vi "파일전송클라이언트.vi"() -> ()   [LabVIEW 2018]
panel:
  out "Sever Connected":bool
  in  "Folder Path":path=path "E:/images" caption="다운로드  경로"
  in  "다운로드":bool
  out "선택한 파일":string
  in  "파일 리스트":i32(listbox)=-1
  in  "업데이트":bool
  out "Echo":string
  in  "정지":bool
  in  "데이터 입력":string
  in  "전송":bool
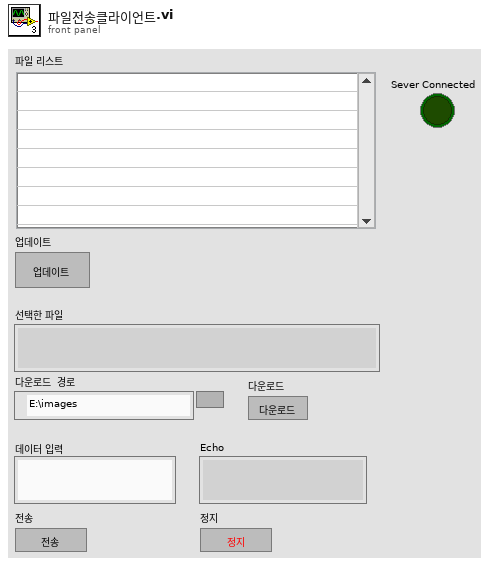
[diagram p1: front panel]
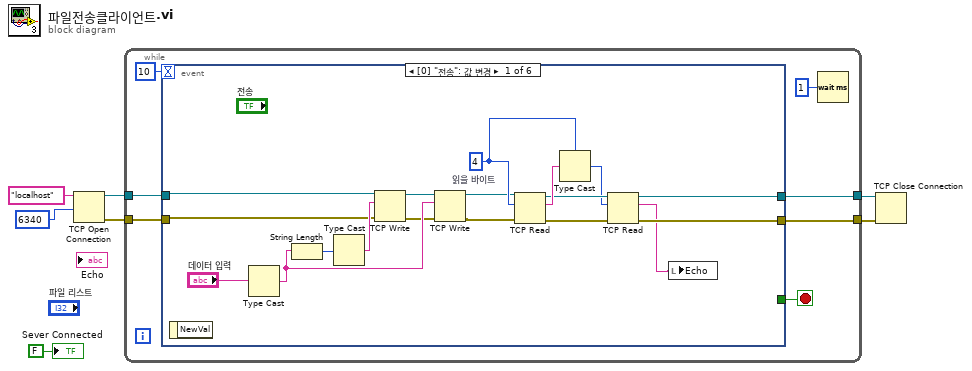
[diagram p0: block diagram]
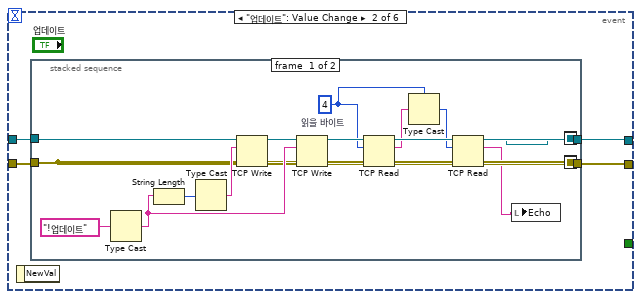
[diagram p2: hidden frame]
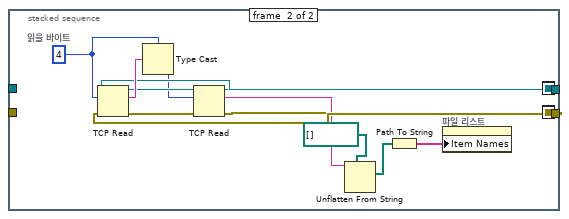
[diagram p3: hidden frame]
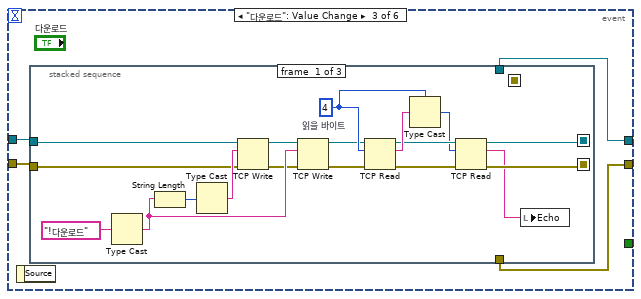
[diagram p4: hidden frame]
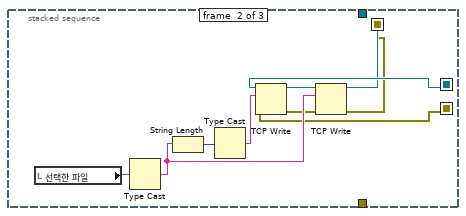
[diagram p5: hidden frame]
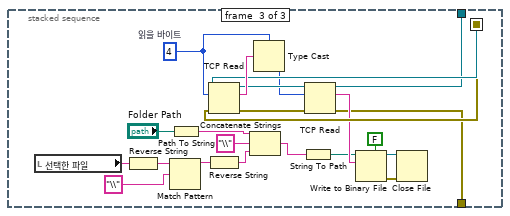
[diagram p6: hidden frame]
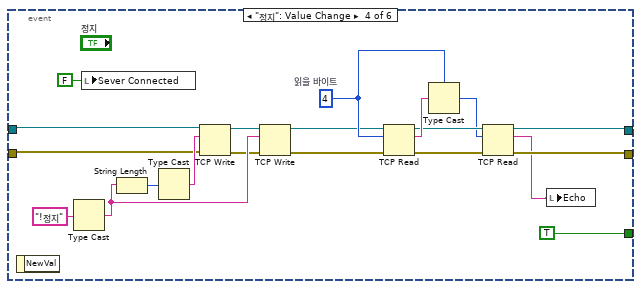
[diagram p7: hidden frame]
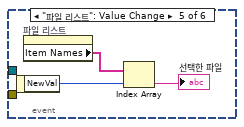
[diagram p8: hidden frame]
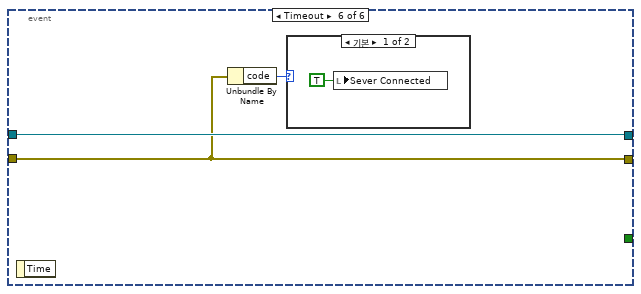
[diagram p9: hidden frame]
diagram:
  n1 = TCP Open Connection(address="localhost" ("주소"), remote port or service name=u16 6340 ("포트")) -> (connection ID=w5:refnum<k5>, error out=w3:errorcluster)  [unwired: 3 in]
  n2 = while {
    tunnel: w5 -> [w14]
    tunnel: [w12] -> w4
    tunnel: w3 -> [w13]
    tunnel: [w11] -> w2
    stop <- w10 stop-if-true
    n3 = event shown="[0] \"전송\": 값 변경" {
      selector: _ -> [_ _ _ _ _ _]
      dyn-events: _ -> [_ _ _ _ _ _]
      timeout: 10 -> [_ _ _ _ _ _]
      tunnel: w14 -> [w26 w36 w71 w137 _ w148]
      tunnel: w13 -> [w25 w35 w70 w136 _ w147]
      tunnel: [w17 w34 w69 w128 _ w148] -> w12
      tunnel: [w16 w33 w68 w127 _ w147] -> w11
      tunnel: [_ _ _ TRUE _ _] -> w10
      event "전송": Value Change {
        w23 = 4  # 읽을 바이트
        n4 = event-data() -> ()  [unwired: 1 in, 1 out]
        n5 = Type Cast(x="데이터 입력") -> (*(type *) &x=w30:string)  [unwired: 1 in]
        n6 = String Length(string=w30) -> (length=w31:i32)
        n7 = Type Cast(x=w31) -> (*(type *) &x=w32:string)  [unwired: 1 in]
        n8 = TCP Write(connection ID=w26, data in=w32, error in (no error)=w25) -> (connection ID out=w29:refnum<k5>, error out=w27:errorcluster)  [unwired: 1 in, 1 out]
        n9 = TCP Write(connection ID=w29, data in=w30, error in (no error)=w27) -> (connection ID out=w22:refnum<k5>, error out=w21:errorcluster)  [unwired: 1 in, 1 out]
        n10 = TCP Read(connection ID=w22, bytes to read=w23, error in (no error)=w21) -> (connection ID out=w19:refnum<k5>, data out=w24:string, error out=w20:errorcluster)  [unwired: 2 in]
        n11 = Type Cast(type=w23, x=w24) -> (*(type *) &x=w18:i32)
        n12 = TCP Read(connection ID=w19, bytes to read=w18, error in (no error)=w20) -> (connection ID out=w17:refnum<k5>, data out=w15:string, error out=w16:errorcluster)  [unwired: 2 in]
        n13 = local write "Echo"(w15) -> ()
      }
      event "업데이트": Value Change {
        n14 = event-data() -> ()  [unwired: 1 in, 1 out]
        n15 = stacked-sequence {
          seq-local: [w49 _] -> [_ w65]
          seq-local: [w48 _] -> [_ w64]
          seq-local: [w40 _] -> [_ _]
          seq-local: [w39 _] -> [_ _]
          tunnel: w36 -> [w49 _]
          tunnel: w35 -> [w48 _]
          tunnel: [_ w58] -> w34
          tunnel: [_ w57] -> w33
          frame #0 {
            w46 = 4  # 읽을 바이트
            n16 = Type Cast(x="!업데이트") -> (*(type *) &x=w52:string)  [unwired: 1 in]
            n17 = String Length(string=w52) -> (length=w53:i32)
            n18 = Type Cast(x=w53) -> (*(type *) &x=w54:string)  [unwired: 1 in]
            n19 = TCP Write(connection ID=w49, data in=w54, error in (no error)=w48) -> (connection ID out=w51:refnum<k5>, error out=w50:errorcluster)  [unwired: 1 in, 1 out]
            n20 = TCP Write(connection ID=w51, data in=w52, error in (no error)=w50) -> (connection ID out=w45:refnum<k5>, error out=w44:errorcluster)  [unwired: 1 in, 1 out]
            n21 = TCP Read(connection ID=w45, bytes to read=w46, error in (no error)=w44) -> (connection ID out=w42:refnum<k5>, data out=w47:string, error out=w43:errorcluster)  [unwired: 2 in]
            n22 = Type Cast(type=w46, x=w47) -> (*(type *) &x=w41:i32)
            n23 = TCP Read(connection ID=w42, bytes to read=w41, error in (no error)=w43) -> (connection ID out=w40:refnum<k5>, data out=w38:string, error out=w39:errorcluster)  [unwired: 2 in]
            n24 = local write "Echo"(w38) -> ()
          }
          frame #1 {
            w66 = 4  # 읽을 바이트
            n25 = TCP Read(connection ID=w65, bytes to read=w66, error in (no error)=w64) -> (connection ID out=w60:refnum<k5>, data out=w67:string, error out=w59:errorcluster)  [unwired: 2 in]
            n26 = Type Cast(type=w66, x=w67) -> (*(type *) &x=w55:i32)
            n27 = TCP Read(connection ID=w60, bytes to read=w55, error in (no error)=w59) -> (connection ID out=w58:refnum<k5>, data out=w62:string, error out=w57:errorcluster)  [unwired: 2 in]
            n28 = Unflatten From String(type=path[] [], binary string=w62) -> (value=w63:path[])  [unwired: 3 in, 2 out]
            n29 = Path To String(path=w63) -> (string=w56:string[])
            n30 = property on="파일 리스트" class="LstBox (엄격한)"("Item Names"=w56) -> ()  [unwired: 2 in, 2 out]
          }
        }
      }
      event "다운로드": Value Change {
        n31 = event-data() -> ()  [unwired: 1 in, 1 out]
        n32 = stacked-sequence {
          seq-local: [w77 _ _] -> [_ w93 _]
          seq-local: [w76 _ _] -> [_ w92 _]
          seq-local: [_ w91 _] -> [_ _ w120]
          seq-local: [_ w90 _] -> [_ _ w119]
          tunnel: w71 -> [w73 _ _]
          tunnel: w70 -> [w72 _ _]
          tunnel: [_ _ w111] -> w69
          tunnel: [_ _ w110] -> w68
          frame #0 {
            w83 = 4  # 읽을 바이트
            n33 = Type Cast(x="!다운로드") -> (*(type *) &x=w87:string)  [unwired: 1 in]
            n34 = String Length(string=w87) -> (length=w88:i32)
            n35 = Type Cast(x=w88) -> (*(type *) &x=w89:string)  [unwired: 1 in]
            n36 = TCP Write(connection ID=w73, data in=w89, error in (no error)=w72) -> (connection ID out=w86:refnum<k5>, error out=w85:errorcluster)  [unwired: 1 in, 1 out]
            n37 = TCP Write(connection ID=w86, data in=w87, error in (no error)=w85) -> (connection ID out=w82:refnum<k5>, error out=w81:errorcluster)  [unwired: 1 in, 1 out]
            n38 = TCP Read(connection ID=w82, bytes to read=w83, error in (no error)=w81) -> (connection ID out=w79:refnum<k5>, data out=w84:string, error out=w80:errorcluster)  [unwired: 2 in]
            n39 = Type Cast(type=w83, x=w84) -> (*(type *) &x=w78:i32)
            n40 = TCP Read(connection ID=w79, bytes to read=w78, error in (no error)=w80) -> (connection ID out=w77:refnum<k5>, data out=w74:string, error out=w76:errorcluster)  [unwired: 2 in]
            n41 = local write "Echo"(w74) -> ()
          }
          frame #1 {
            n42 = local read "선택한 파일"() -> (w94:string)
            n43 = Type Cast(x=w94) -> (*(type *) &x=w97:string)  [unwired: 1 in]
            n44 = String Length(string=w97) -> (length=w98:i32)
            n45 = Type Cast(x=w98) -> (*(type *) &x=w99:string)  [unwired: 1 in]
            n46 = TCP Write(connection ID=w93, data in=w99, error in (no error)=w92) -> (connection ID out=w96:refnum<k5>, error out=w95:errorcluster)  [unwired: 1 in, 1 out]
            n47 = TCP Write(connection ID=w96, data in=w97, error in (no error)=w95) -> (connection ID out=w91:refnum<k5>, error out=w90:errorcluster)  [unwired: 1 in, 1 out]
          }
          frame #2 {
            w121 = 4  # 읽을 바이트
            n48 = local read "선택한 파일"() -> (w107:string)
            n49 = Reverse String(1:w107) -> (0:w106:string)
            n50 = Match Pattern(string=w106, regular expression="\\" ("정규식")) -> (before substring=w108:string)  [unwired: 1 in, 3 out]
            n51 = Path To String(path="Folder Path") -> (string=w100:string)
            n52 = TCP Read(connection ID=w120, bytes to read=w121, error in (no error)=w119) -> (connection ID out=w118:refnum<k5>, data out=w122:string, error out=w117:errorcluster)  [unwired: 2 in]
            n53 = Reverse String(1:w108) -> (0:w104:string)
            n54 = Concatenate Strings(w100, "\\" ("문자열"), w104) -> (w101:string)
            n55 = Type Cast(type=w121, x=w122) -> (*(type *) &x=w116:i32)
            n56 = String To Path(string=w101) -> (path=w102:path)
            n57 = TCP Read(connection ID=w118, bytes to read=w116, error in (no error)=w117) -> (connection ID out=w111:refnum<k5>, data out=w112:string, error out=w110:errorcluster)  [unwired: 2 in]
            n58 = Write to Binary File(file (use dialog)=w102, data=w112, 5:FALSE ("배열 또는 문자열 크기를 앞에 추가? (참)")) -> (refnum out=w114:refnum<file>, error out=w115:errorcluster)  [unwired: 3 in, 1 out]
            n59 = Close File(refnum=w114, error in=w115) -> ()  [unwired: 2 out]
          }
        }
      }
      event "정지": Value Change {
        w134 = 4  # 읽을 바이트
        n60 = event-data() -> ()  [unwired: 1 in, 1 out]
        n61 = Type Cast(x="!정지") -> (*(type *) &x=w140:string)  [unwired: 1 in]
        n62 = local write "Sever Connected"(FALSE ("Sever Connected")) -> ()
        n63 = String Length(string=w140) -> (length=w141:i32)
        n64 = Type Cast(x=w141) -> (*(type *) &x=w142:string)  [unwired: 1 in]
        n65 = TCP Write(connection ID=w137, data in=w142, error in (no error)=w136) -> (connection ID out=w139:refnum<k5>, error out=w138:errorcluster)  [unwired: 1 in, 1 out]
        n66 = TCP Write(connection ID=w139, data in=w140, error in (no error)=w138) -> (connection ID out=w133:refnum<k5>, error out=w132:errorcluster)  [unwired: 1 in, 1 out]
        n67 = TCP Read(connection ID=w133, bytes to read=w134, error in (no error)=w132) -> (connection ID out=w130:refnum<k5>, data out=w135:string, error out=w131:errorcluster)  [unwired: 2 in]
        n68 = Type Cast(type=w134, x=w135) -> (*(type *) &x=w129:i32)
        n69 = TCP Read(connection ID=w130, bytes to read=w129, error in (no error)=w131) -> (connection ID out=w128:refnum<k5>, data out=w125:string, error out=w127:errorcluster)  [unwired: 2 in]
        n70 = local write "Echo"(w125) -> ()
      }
      event "파일 리스트": Value Change {
        n71 = event-data() -> ("NewVal"=w144:i32)  [unwired: 1 in]
        n72 = property on="파일 리스트" class="LstBox (엄격한)"() -> ("Item Names"=w143:string[])  [unwired: 2 in, 2 out]
        n73 = Index Array(array=w143, index=w144) -> (element=→"선택한 파일":string)
      }
      event Timeout {
        n74 = event-data() -> ()  [unwired: 1 in, 1 out]
        n75 = Unbundle By Name(w147) -> ("code"=w146:i32)
        n76 = case shown="기본" w146 {
          frame Default {
            n77 = local write "Sever Connected"(TRUE ("Sever Connected")) -> ()
          }
          frame 63 {
          }
        }
      }
    }
    n78 = Wait (ms)(milliseconds to wait=u32 1 ("대기 시간 (ms)")) -> ()  [unwired: 1 out]
  }
  n79 = TCP Close Connection(connection ID=w4, error in (no error)=w2) -> ()  [unwired: 1 in, 2 out]
  "Sever Connected" <- FALSE ("Sever Connected")
